vi "SQL_6133_data_insert.vi"(0 "数据":T1={"时间"=timestamp(3515985789.500352 s since 1904-01-01), "声发射"=array[32000 elements], "电涡流1"=array[32000 elements], "电涡流2"=array[32000 elements], "电涡流3"=array[32000 elements], "电涡流4"=array[32000 elements], "电涡流5"=array[32000 elements], "加速度1"=array[80000 elements], "加速度2"=array[80000 elements]}) -> (7 "error out":errorcluster, 8 "数据插入时间ms":u32)   [LabVIEW 2014]
uses:
  <vilib>/addons/database/Connection.llb/DB Tools Open Connec (String).vi
  <vilib>/addons/database/Connection.llb/Conn Execute.vi
  <vilib>/addons/database/Recordset.llb/Rec Destroy - Connection.vi
  <vilib>/addons/database/NI_Database_API.lvlib
panel:
  out "x-y":u32
  out "毫秒计时值 2":u32
  out "毫秒计时值":u32
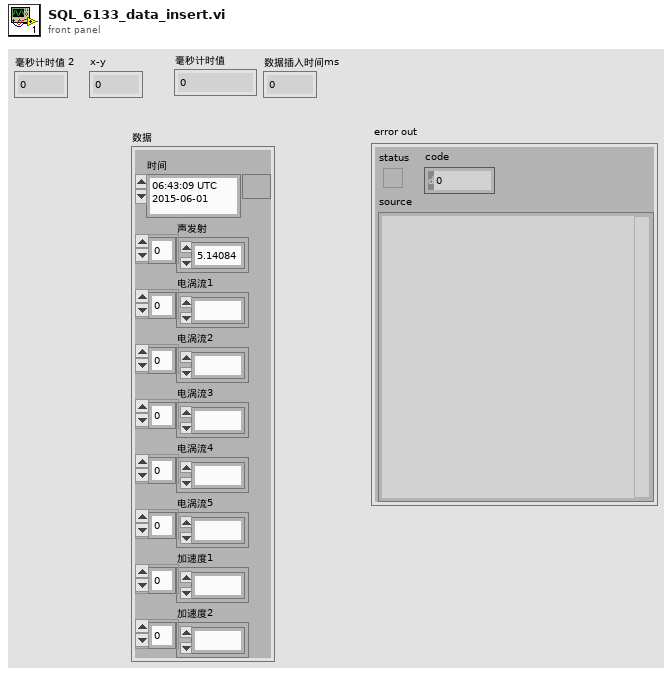
[diagram p1: front panel]
types:
  T1 = cluster{"时间":timestamp, "声发射":sgl[], "电涡流1":sgl[], "电涡流2":sgl[], "电涡流3":sgl[], "电涡流4":sgl[], "电涡流5":sgl[], "加速度1":sgl[], "加速度2":sgl[]}
  T2 = cluster{string, string, string, string, string, string, string, string}
  T3 = typedef "NI_Database_API.lvlib/Conn ObjectReference.ctl" = refnum<k1>
  T4 = typedef "NI_Database_API.lvlib/Rec ObjectReference.ctl" = refnum<k1>
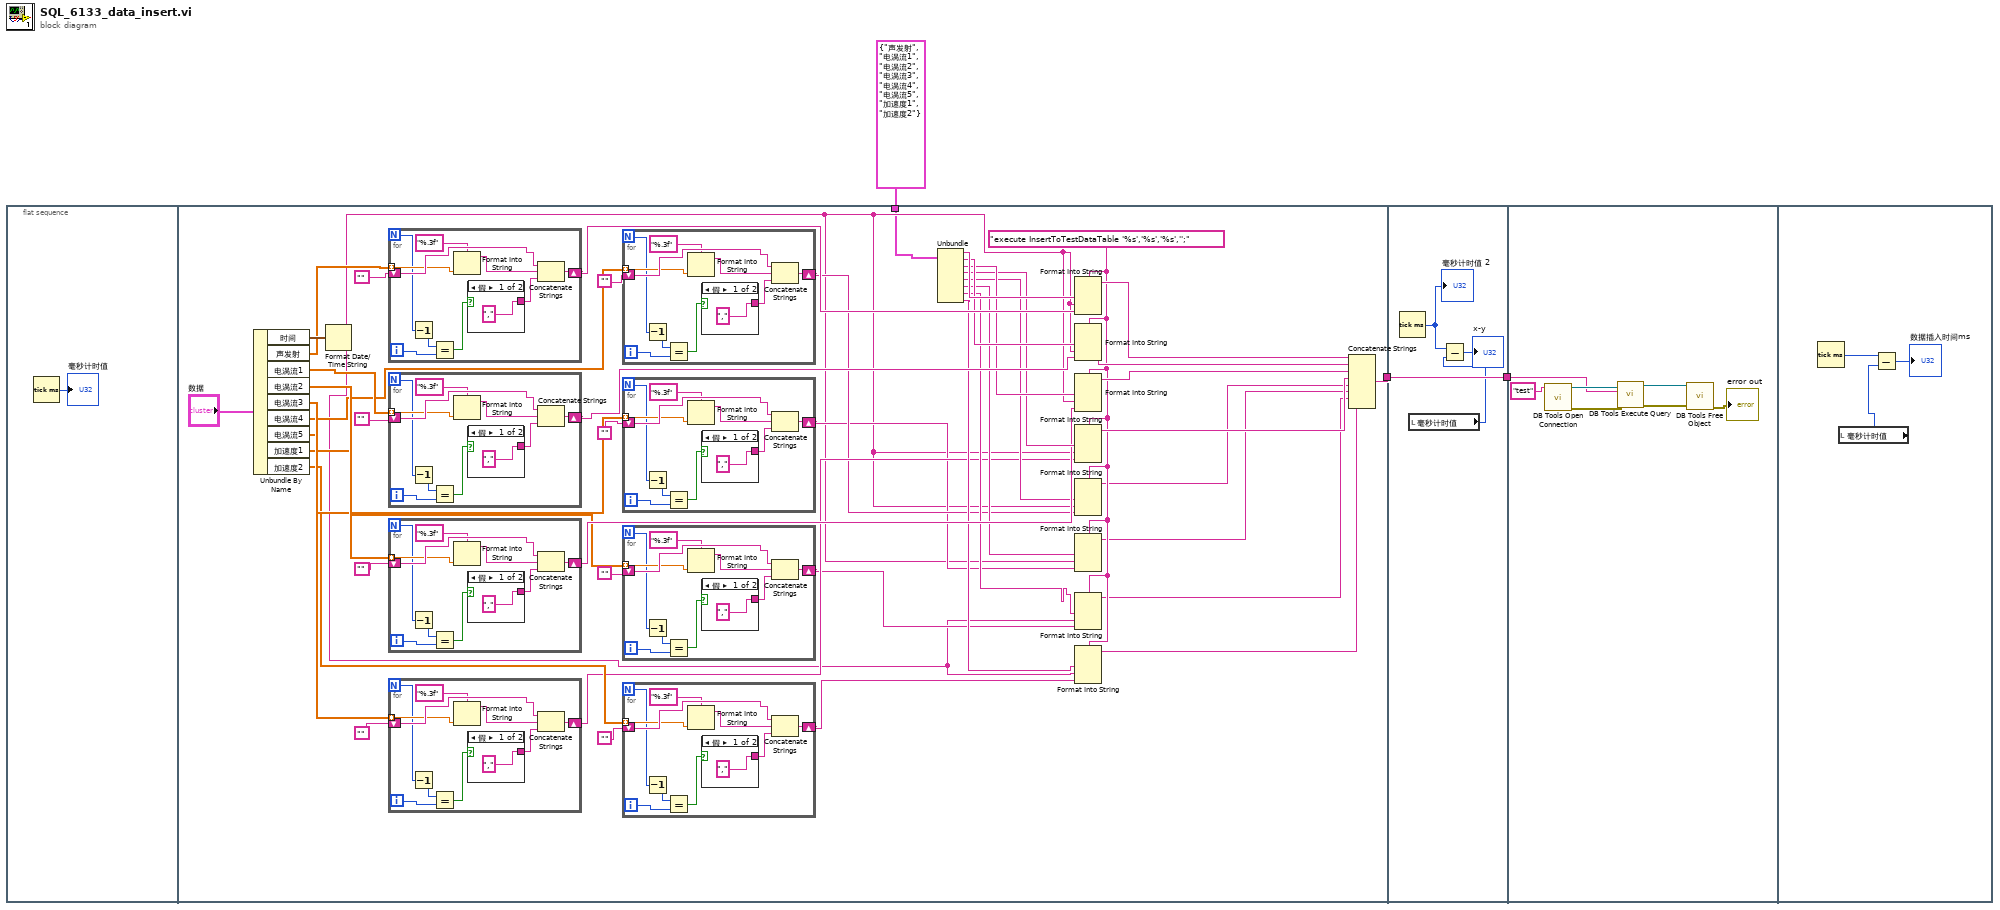
[diagram p0: block diagram]
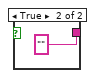
[diagram p2: hidden frame]
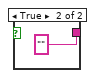
[diagram p3: hidden frame]
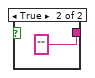
[diagram p4: hidden frame]
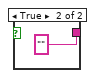
[diagram p5: hidden frame]
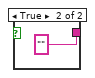
[diagram p6: hidden frame]
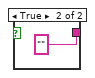
[diagram p7: hidden frame]
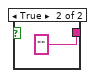
[diagram p8: hidden frame]
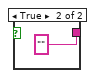
[diagram p9: hidden frame]
diagram:
  n1 = flat-sequence {
    tunnel: [w50] -> w3
    tunnel: T2 {"声发射", "电涡流1", "电涡流2", "电涡流3", "电涡流4", "电涡流5", "加速度1", "加速度2"} ("通道名") -> [w5]
    tunnel: w3 -> [w150]
    tunnel: [w150] -> w2
    tunnel: w2 -> [w151]
    frame #0 {
      n2 = Tick Count (ms)() -> (millisecond timer value=→"毫秒计时值":u32)
    }
    frame #1 {
      w16 = "execute InsertToTestDataTable '%s','%s','%s','';"
      n3 = Unbundle By Name("数据") -> ("时间"=w49:timestamp, "声发射"=w44:sgl[], "电涡流1"=w43:sgl[], "电涡流2"=w41:sgl[], "电涡流3"=w39:sgl[], "电涡流4"=w28:sgl[], "电涡流5"=w27:sgl[], "加速度1"=w26:sgl[], "加速度2"=w25:sgl[])
      n4 = Format Date/Time String(seconds (now)=w49) -> (date/time string=w10:string)  [unwired: 2 in]
      n5 = for "For循环" {
        N -> [w137]
        tunnel: w44 -> [w142] mode=indexing
        shift-right: [w143] -> w46
        shift-left: "" -> [w144]
        i -> [w139]
        n6 = Decrement(x=w137) -> (x-1=w138:i32)
        n7 = Equal?(x=w138, y=w139) -> (x = y?=w136:bool)
        n8 = Format Into String(format string="%.3f", w142) -> (resulting string=w141:string)  [unwired: 2 in, 1 out]
        n9 = case shown="假" w136 {
          tunnel: ["," ""] -> w135
          frame False {
          }
          frame True {
          }
        }
        n10 = Concatenate Strings(w144, w141, w135) -> (w143:string)
      }
      n11 = for "For循环" {
        N -> [w125]
        tunnel: w43 -> [w130] mode=indexing
        shift-right: [w131] -> w37
        shift-left: "" -> [w132]
        i -> [w127]
        n12 = Decrement(x=w125) -> (x-1=w126:i32)
        n13 = Equal?(x=w126, y=w127) -> (x = y?=w124:bool)
        n14 = Format Into String(format string="%.3f", w130) -> (resulting string=w129:string)  [unwired: 2 in, 1 out]
        n15 = case shown="假" w124 {
          tunnel: ["," ""] -> w123
          frame False {
          }
          frame True {
          }
        }
        n16 = Concatenate Strings(w132, w129, w123) -> (w131:string)
      }
      n17 = for "For循环" {
        N -> [w113]
        tunnel: w41 -> [w118] mode=indexing
        shift-right: [w119] -> w32
        shift-left: "" -> [w120]
        i -> [w115]
        n18 = Decrement(x=w113) -> (x-1=w114:i32)
        n19 = Equal?(x=w114, y=w115) -> (x = y?=w112:bool)
        n20 = Format Into String(format string="%.3f", w118) -> (resulting string=w117:string)  [unwired: 2 in, 1 out]
        n21 = case shown="假" w112 {
          tunnel: ["," ""] -> w111
          frame False {
          }
          frame True {
          }
        }
        n22 = Concatenate Strings(w120, w117, w111) -> (w119:string)
      }
      n23 = for "For循环" {
        N -> [w101]
        tunnel: w39 -> [w106] mode=indexing
        shift-right: [w107] -> w15
        shift-left: "" -> [w108]
        i -> [w103]
        n24 = Decrement(x=w101) -> (x-1=w102:i32)
        n25 = Equal?(x=w102, y=w103) -> (x = y?=w100:bool)
        n26 = Format Into String(format string="%.3f", w106) -> (resulting string=w105:string)  [unwired: 2 in, 1 out]
        n27 = case shown="假" w100 {
          tunnel: ["," ""] -> w99
          frame False {
          }
          frame True {
          }
        }
        n28 = Concatenate Strings(w108, w105, w99) -> (w107:string)
      }
      n29 = for "For循环" {
        N -> [w89]
        tunnel: w28 -> [w94] mode=indexing
        shift-right: [w95] -> w14
        shift-left: "" -> [w96]
        i -> [w91]
        n30 = Decrement(x=w89) -> (x-1=w90:i32)
        n31 = Equal?(x=w90, y=w91) -> (x = y?=w88:bool)
        n32 = Format Into String(format string="%.3f", w94) -> (resulting string=w93:string)  [unwired: 2 in, 1 out]
        n33 = case shown="假" w88 {
          tunnel: ["," ""] -> w87
          frame False {
          }
          frame True {
          }
        }
        n34 = Concatenate Strings(w96, w93, w87) -> (w95:string)
      }
      n35 = for "For循环" {
        N -> [w77]
        tunnel: w27 -> [w82] mode=indexing
        shift-right: [w83] -> w13
        shift-left: "" -> [w84]
        i -> [w79]
        n36 = Decrement(x=w77) -> (x-1=w78:i32)
        n37 = Equal?(x=w78, y=w79) -> (x = y?=w76:bool)
        n38 = Format Into String(format string="%.3f", w82) -> (resulting string=w81:string)  [unwired: 2 in, 1 out]
        n39 = case shown="假" w76 {
          tunnel: ["," ""] -> w75
          frame False {
          }
          frame True {
          }
        }
        n40 = Concatenate Strings(w84, w81, w75) -> (w83:string)
      }
      n41 = for "For循环" {
        N -> [w65]
        tunnel: w26 -> [w70] mode=indexing
        shift-right: [w71] -> w12
        shift-left: "" -> [w72]
        i -> [w67]
        n42 = Decrement(x=w65) -> (x-1=w66:i32)
        n43 = Equal?(x=w66, y=w67) -> (x = y?=w64:bool)
        n44 = Format Into String(format string="%.3f", w70) -> (resulting string=w69:string)  [unwired: 2 in, 1 out]
        n45 = case shown="假" w64 {
          tunnel: ["," ""] -> w63
          frame False {
          }
          frame True {
          }
        }
        n46 = Concatenate Strings(w72, w69, w63) -> (w71:string)
      }
      n47 = for "For循环" {
        N -> [w53]
        tunnel: w25 -> [w58] mode=indexing
        shift-right: [w59] -> w11
        shift-left: "" -> [w60]
        i -> [w55]
        n48 = Decrement(x=w53) -> (x-1=w54:i32)
        n49 = Equal?(x=w54, y=w55) -> (x = y?=w52:bool)
        n50 = Format Into String(format string="%.3f", w58) -> (resulting string=w57:string)  [unwired: 2 in, 1 out]
        n51 = case shown="假" w52 {
          tunnel: ["," ""] -> w51
          frame False {
          }
          frame True {
          }
        }
        n52 = Concatenate Strings(w60, w57, w51) -> (w59:string)
      }
      n53 = Unbundle(w5) -> (w36:string, w35:string, w34:string, w33:string, w20:string, w19:string, w18:string, w17:string)
      n54 = Format Into String ("格式化写入字符串")(format string=w16, w36, w10, w46) -> (resulting string=w48:string)  [unwired: 2 in, 1 out]
      n55 = Format Into String ("格式化写入字符串")(format string=w16, w35, w10, w37) -> (resulting string=w31:string)  [unwired: 2 in, 1 out]
      n56 = Format Into String ("格式化写入字符串")(format string=w16, w34, w10, w32) -> (resulting string=w30:string)  [unwired: 2 in, 1 out]
      n57 = Format Into String ("格式化写入字符串")(format string=w16, w33, w10, w15) -> (resulting string=w29:string)  [unwired: 2 in, 1 out]
      n58 = Format Into String ("格式化写入字符串")(format string=w16, w20, w10, w14) -> (resulting string=w9:string)  [unwired: 2 in, 1 out]
      n59 = Format Into String ("格式化写入字符串")(format string=w16, w19, w10, w13) -> (resulting string=w8:string)  [unwired: 2 in, 1 out]
      n60 = Format Into String ("格式化写入字符串")(format string=w16, w18, w10, w12) -> (resulting string=w7:string)  [unwired: 2 in, 1 out]
      n61 = Format Into String ("格式化写入字符串")(format string=w16, w17, w10, w11) -> (resulting string=w6:string)  [unwired: 2 in, 1 out]
      n62 = Concatenate Strings ("连接字符串")(w48, w31, w30, w29, w9, w8, w7, w6) -> (w50:string)
    }
    frame #2 {
      n63 = Tick Count (ms)() -> (millisecond timer value=w149:u32)
      "毫秒计时值 2" <- w149
      n64 = local read "毫秒计时值"() -> (w148:u32)
      n65 = Subtract(x=w149, y=w148) -> (x-y=→"x-y":u32)
    }
    frame #3 {
      n66 = call-poly <vilib>:"DB Tools Open Connection.vi"("connection information"="test") -> ("error out"=w157:errorcluster, "connection reference"=w156:T3)  [unwired: 7 in]
      n67 = call-poly <vilib>:"DB Tools Execute Query.vi"("error in (no error)"=w157, "SQL query"=w151, "connection reference"=w156) -> ("error out"=w154:errorcluster, "recordset reference"=w153:T4)  [unwired: 5 in]
      n68 = call-poly <vilib>:"DB Tools Free Object.vi"("error in (no error)"=w154, "recordset reference"=w153) -> ("error out"=→"error out":errorcluster)  [unwired: 8 in, 1 out]
    }
    frame #4 {
      n69 = Tick Count (ms)() -> (millisecond timer value=w160:u32)
      n70 = local read "毫秒计时值"() -> (w158:u32)
      n71 = Subtract(x=w160, y=w158) -> (x-y=→"数据插入时间ms":u32)
    }
  }
